vi "Vision Research Phantom Series PhInt PhFlipsPAR.vi"(2 "pPixel in":u16[](array[numeric]), 5 "Error In (no error)":errorcluster, 7 "BITMAPINFOHEADER":T5, 9 "IMPROCOPTIONS":T1 {"FilterCode" items=["PREWITT_3X3_V"=1, "PREWITT_3X3_H"=2, "SOBEL_3X3_V"=3, "SOBEL_3X3_H"=4, "LAPLACIAN_3X3"=5, "LAPLACIAN_5X5"=6, "GAUSSIAN_3X3"=7, "GAUSSIAN_5X5"=8, "HIPASS_3x3"=9, "HIPASS_5x5"=10, "SHARPEN_3X3"=11, "USERFILTER"=-1]; "Rotate" min=-90 max=90 step=1; "Saturation" min=-100 max=100 step=1; "Contrast" min=-100 max=100 step=1; "Bright" min=-100 max=100 step=1}) -> (16 "pPixel":u16[](array[numeric]), 19 "Error Out":errorcluster)   [LabVIEW 2013, in "VRI.lvlib"]
doc: "PhInt.dll\n\nPhFlipsPAR\nPhFlipsPAR(int Width, int Height, int BitCount, unsigned char * pPixel, int bFlipH, int bFlipV);\n\nParameters Description\nWidth Image width\nHeight Image height\nBitCount Bits per pixel\npPixel Pixel array pointer\nbFlipV Flip Vertical if TRUE\nbFlipH Flip Horizontal if TRUE\nReturn Void\nComments A replacement for LabView of the PhMakeColor function\n\nWritten by:\nBLOOMY CONTROLS, INC\nWINDSOR, CT 06095, USA\n860-298-9925\nwww.bloomy.com\nV1.0.0\nMay, 2004"
uses:
  VRI.lvlib
  _Type Defs/BITMAPINFOHEADER.ctl
  _Type Defs/PhInt IMPROCOPTIONS.ctl
  _Type Defs/PhInt WBGAIN.ctl
  _Type Defs/FilterCode.ctl
  _Type Defs/IMFILTER.ctl
  Phantom DLLs/PhInt.dll
panel:
  # "For instructions on the use of this VI, press Ctrl+H to display the help window and move the mouse over the icon, controls, and indicators"
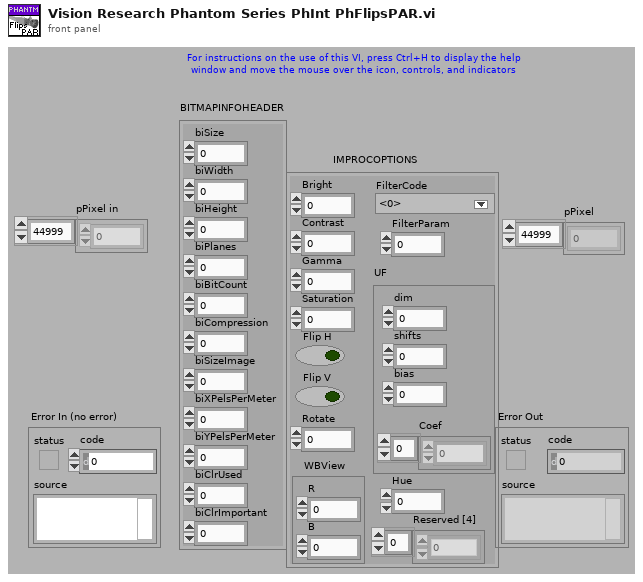
[diagram p1: front panel]
types:
  T1 = typedef "VRI.lvlib/PhInt IMPROCOPTIONS.ctl" = cluster{"Bright":i32, "Contrast":i32, "Gamma":sgl, "Saturation":i32, "Flip H":bool, "Flip V":bool, "Rotate":i32, "WBView":T2, "FilterCode":T3, "FilterParam":i32, "UF":T4, "Hue":i32, "Reserved [4]":i32[]}
  T2 = typedef "VRI.lvlib/PhInt WBGAIN.ctl" = cluster{"R":sgl, "B":sgl}
  T3 = typedef "VRI.lvlib/FilterCode.ctl" = i32
  T4 = typedef "VRI.lvlib/IMFILTER.ctl" = cluster{"dim":i32, "shifts":i32, "bias":i32, "Coef":i32[]}
  T5 = typedef "VRI.lvlib/BITMAPINFOHEADER.ctl" = cluster{"biSize":u32, "biWidth":i32, "biHeight":i32, "biPlanes":u16, "biBitCount":u16, "biCompression":u32, "biSizeImage":u32, "biXPelsPerMeter":i32, "biYPelsPerMeter":i32, "biClrUsed":u32, "biClrImportant":u32}
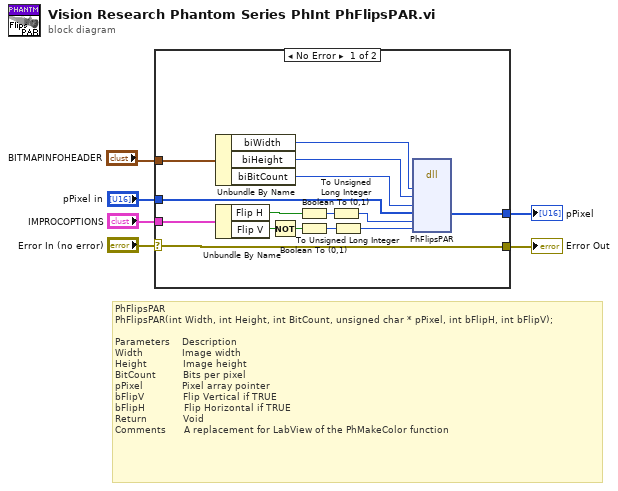
[diagram p0: block diagram]
diagram:
  # "PhFlipsPAR\nPhFlipsPAR(int Width, int Height, int BitCount, unsigned char * pPixel, int bFlipH, int bFlipV);\n\nParameters    Description\nWidth             Image width\nHeight            Image height\nBitCount         Bits per pixel\npPixel             Pixel array pointer\nbFlipV             Flip Vertical if TRUE\nbFlipH             Flip Horizontal if TRUE\nReturn            Void\nComments      A replacement for LabView of the PhMakeColor function"
  n1 = case shown="No Error" "Error In (no error)" {
    selector: "Error In (no error)" -> [w21 w22]
    tunnel: [w21 w22] -> w5
    tunnel: "BITMAPINFOHEADER" -> [w20 _]
    tunnel: [w19 _] -> w4
    tunnel: "IMPROCOPTIONS" -> [w18 _]
    tunnel: "pPixel in" -> [w17 _]
    frame No Error {
      n2 = Unbundle By Name(w20) -> ("biWidth"=w16:i32, "biHeight"=w15:i32, "biBitCount"=w14:u16)
      n3 = Unbundle By Name(w18) -> ("Flip H"=w13:bool, "Flip V"=w12:bool)
      n4 = Not(x=w12) -> (.not. x?=w7:bool)
      n5 = Boolean To (0,1)(Boolean=w13) -> (0, 1=w11:i16)
      n6 = Boolean To (0,1)(Boolean=w7) -> (0, 1=w10:i16)
      n7 = To Unsigned Long Integer(number=w11) -> (unsigned 32bit integer=w9:u32)
      n8 = To Unsigned Long Integer(number=w10) -> (unsigned 32bit integer=w8:u32)
      n9 = dll-call lib="C:/Projects/SDK/32-bit/Vision Research Phantom Series Labview Driver/Phantom DLLs/PhInt.dll" fn="PhFlipsPAR"("Width"=w16, "Height"=w15, "BitCount"=w14, "pPixel"=w17, "FlipV"=w9, "FlipH"=w8) -> ("pPixel"=w19:u16[])  [unwired: 8 in, 3 out]
    }
    frame Error {
    }
  }
  "Error Out" <- w5
  "pPixel" <- w4
